vi "Main.vi"() -> ()   [LabVIEW 2024]
uses:
  <instrlib>/niScope/Acquire/Fetch/niScope Multi Fetch WDT.vi
panel:
  in  "Tab Control":T1(tab)
  in  "Scopes":refnum<k15>[](array[refnum])=["SCOPE1", "SCOPE2"] caption="resource name"
  in  "FGENs":refnum<k15>[](array[refnum])=["FGEN1", "FGEN2"] caption="Resource Name"
  out "Preparing NI-TClk":bool
  in  "Synchronization Method":enum32{"Manual", "T-Clk"}(radio)
  out "Phase Difference @ 10 MHz":dbl format="%#.2g °"
  out "Timing Diagram":digitalwaveform[](graph)
  in  "Stop":bool
  out "Waveform Graph":waveform(dbl)[](graph)
  # "Using NI-TClk to Align Sample Clocks and Improve Synchronization"
  # "Acquired Data"
  # "Time from Trigger to First Sample"
  # "Box Instruments: Cabled Connectivity"
  # "PXI: Integrated Connectivity"
  # "Hardware Configuration"
  # "Synchronization Method"
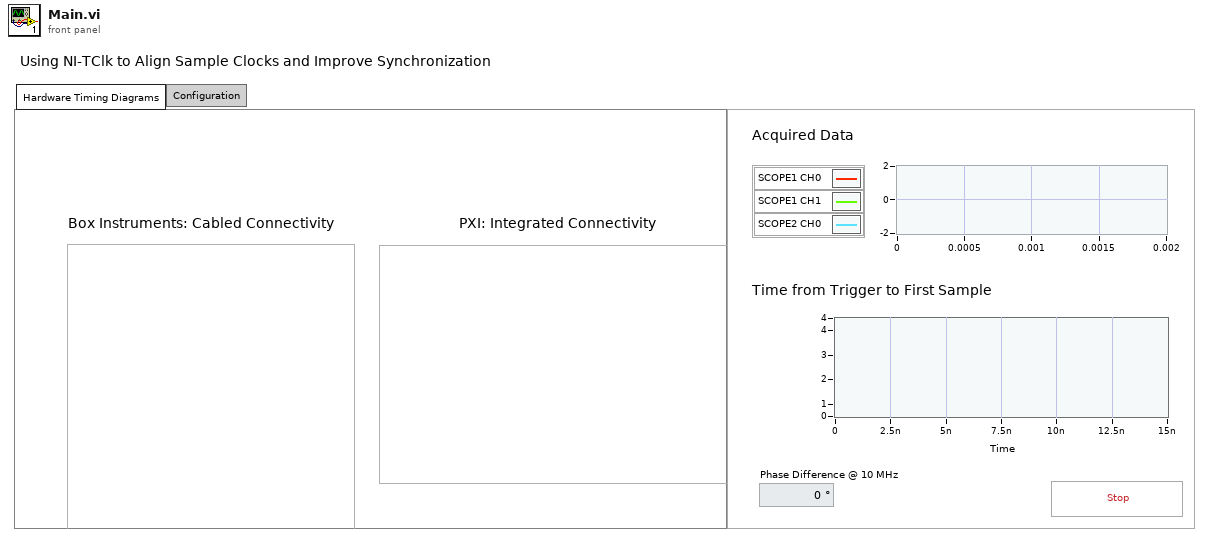
[diagram p1: front panel]
types:
  T1 = enum32{"Hardware Timing Diagrams", "Configuration"}
  T2 = cluster{"actualSamples":i32, "absoluteInitialX":dbl, "relativeInitialX":dbl, "xIncrement":dbl, "offset":dbl, "gain":dbl, "reserved1":dbl, "reserved2":dbl}[]
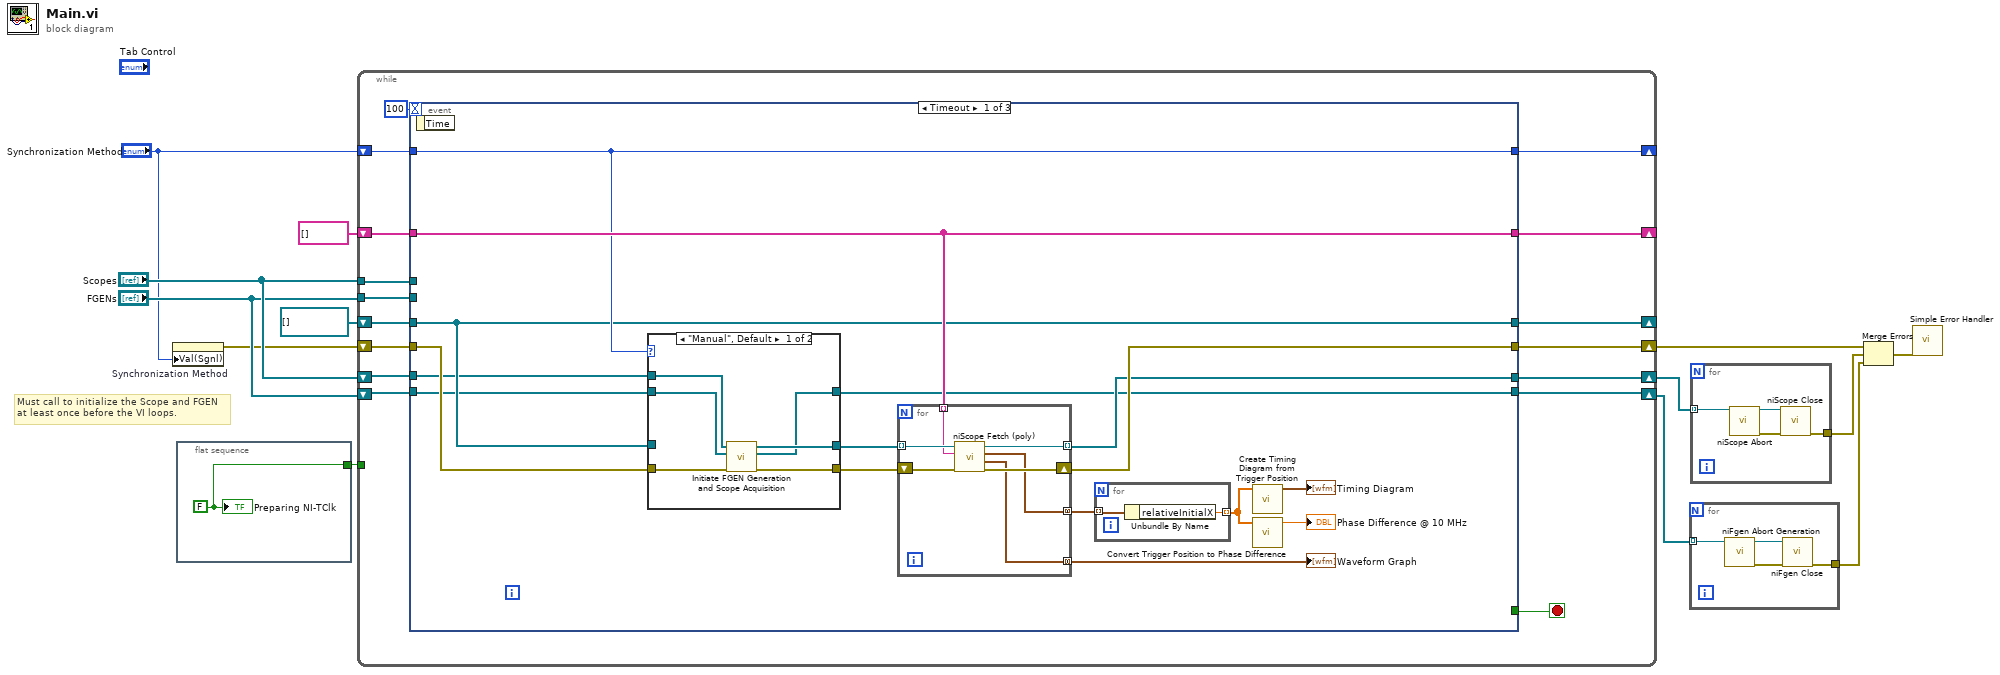
[diagram p0: block diagram]
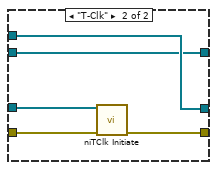
[diagram p2: hidden frame]
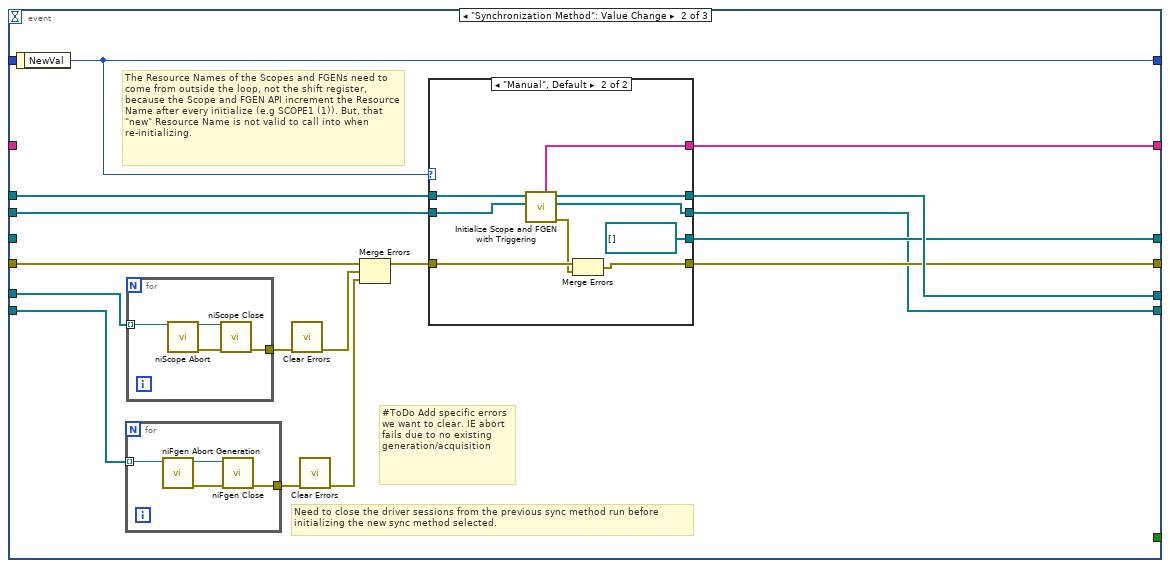
[diagram p3: hidden frame]
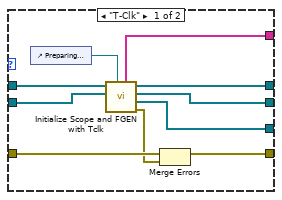
[diagram p4: hidden frame]
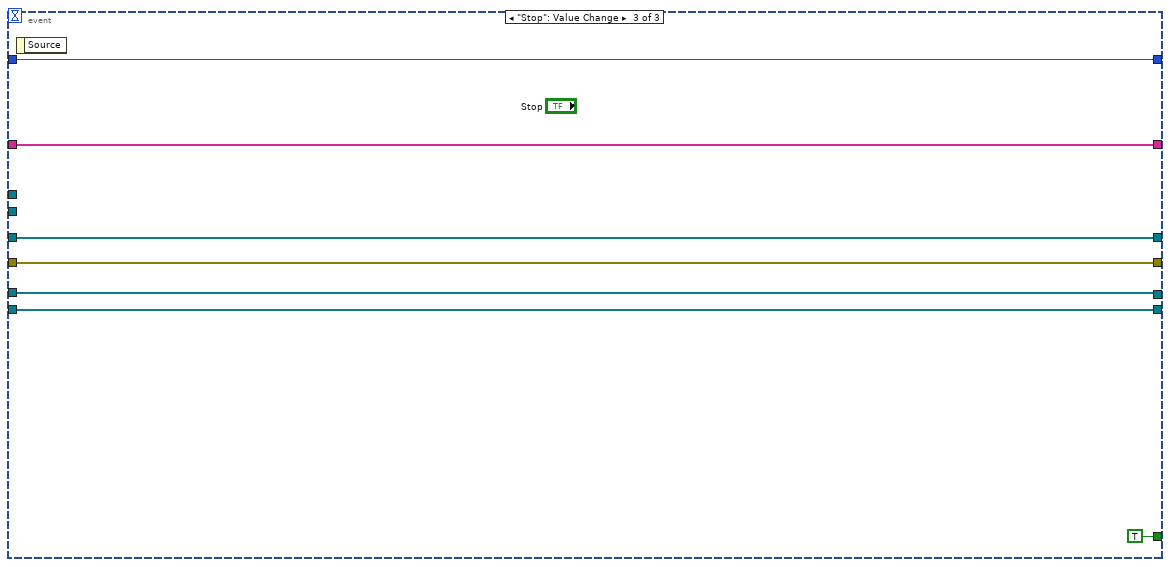
[diagram p5: hidden frame]
diagram:
  # "Must call to initialize the Scope and FGEN \nat least once before the VI loops."
  n1 = property on="Synchronization Method" class="RadioBtnsControl (strict)"("Val(Sgnl)"="Synchronization Method") -> (error out=w8:errorcluster)  [unwired: 2 in, 1 out]
  n2 = flat-sequence {
    tunnel: [w14] -> w9
    frame #0 {
      w14 = FALSE ("Preparing T-Clk")
      "Preparing NI-TClk" <- w14
    }
  }
  n3 = while {
    shift-right: [w28] -> _
    shift-left: "Synchronization Method" -> [w27]
    shift-right: [w24] -> _
    shift-left: string[] [] ("scope channels") -> [w20]
    shift-right: [w23] -> _
    shift-left: refnum<k20>[] [] ("Tclk Refs Array") -> [w21]
    shift-right: [w19] -> w5
    shift-left: w8 -> [w22]
    shift-right: [w16] -> w7
    shift-left: "Scopes" -> [w18]
    shift-right: [w15] -> w6
    shift-left: "FGENs" -> [w17]
    tunnel: w9 -> [_]
    tunnel: "Scopes" -> [w26]
    tunnel: "FGENs" -> [w25]
    stop <- w29 stop-if-true
    n4 = event shown="[0] Timeout" {
      selector: _ -> [_ _ _]
      dyn-events: _ -> [_ _ _]
      timeout: 100 -> [_ _ _]
      tunnel: [_ _ TRUE] -> w29
      tunnel: w25 -> [_ w77 _]
      tunnel: [w35 w82 w112] -> w28
      tunnel: w27 -> [w35 _ w112]
      tunnel: w26 -> [_ w78 _]
      tunnel: [w37 w81 w111] -> w16
      tunnel: [w36 w80 w115] -> w24
      tunnel: [w34 w79 w114] -> w23
      tunnel: w22 -> [w43 w74 w113]
      tunnel: w21 -> [w34 _ w114]
      tunnel: w20 -> [w36 _ w115]
      tunnel: [w38 w75 w113] -> w19
      tunnel: w18 -> [w33 w68 w111]
      tunnel: w17 -> [w32 w67 w110]
      tunnel: [w31 w69 w110] -> w15
      event Timeout {
        n5 = event-data() -> ()  [unwired: 1 in, 1 out]
        n6 = case shown="\"Manual\", Default" w35 {
          tunnel: [w49 w57] -> w42
          tunnel: w34 -> [_ w56]
          tunnel: w43 -> [w52 w55]
          tunnel: w33 -> [w48 w54]
          tunnel: w32 -> [w51 w53]
          tunnel: [w50 w54] -> w40
          tunnel: [w47 w53] -> w31
          frame "Manual", Default {
            n7 = call "Initiate FGEN Generation and Scope Acquisition.vi"("error in (no error)"=w52, "FGEN Resources in"=w51, "Scope Resources in"=w48) -> ("error out"=w49:errorcluster, "FGEN Resources out"=w47:refnum<k15>[], "Scope Resources out"=w50:refnum<k15>[])  [unwired: 6 in]
          }
          frame "T-Clk" {
            n8 = call <instrlib>:"niTClk Initiate.vi"("error in (no error)"=w55, "sessions"=w56) -> ("error out"=w57:errorcluster)  [unwired: 8 in, 1 out]
          }
        }
        n9 = for {
          tunnel: [w62] -> w44 mode=concatenating
          tunnel: [w61] -> w41 mode=concatenating
          shift-right: [w64] -> w38
          shift-left: w42 -> [w63]
          tunnel: w40 -> [w60] mode=indexing
          tunnel: w36 -> [w59] mode=indexing
          tunnel: [w58] -> w37 mode=indexing
          n10 = call-poly <instrlib>:"niScope Fetch (poly).vi"("error in"=w63, "channels"=w59, "instrument handle"=w60) -> ("error out"=w64:errorcluster, "wfm"=w62:waveform(dbl)[], "wfm info"=w61:T2, "instrument handle out"=w58:refnum<k15>)  [unwired: 5 in]
        }
        "Waveform Graph" <- w44
        n11 = for {
          tunnel: w41 -> [w66] mode=indexing
          tunnel: [w65] -> w39 mode=indexing
          n12 = Unbundle By Name(w66) -> ("relativeInitialX"=w65:dbl)
        }
        n13 = call "Create Timing Diagram from Trigger Position.vi"("Relative Trigger Position in"=w39) -> ("Timing Diagram"=→"Timing Diagram":digitalwaveform[])  [unwired: 10 in]
        n14 = call "Convert Trigger Position to Phase Difference.vi"("Relative Trigger Position in"=w39) -> ("Phase Difference"=→"Phase Difference @ 10 MHz":dbl)  [unwired: 10 in]
      }
      event "Synchronization Method": Value Change {
        # "The Resource Names of the Scopes and FGENs need to come from outside the loop, not the shift register, because the Scope and FGEN API increment the Resource Name after every initialize (e.g SCOPE1 (1)). But, that \"new\" Resource Name is not valid to call into when re-initializing."
        # "Need to close the driver sessions from the previous sync method run before\ninitializing the new sync method selected."
        # "#ToDo Add specific errors we want to clear. IE abort fails due to no existing generation/acquisition"
        n15 = event-data() -> ("NewVal"=w82:enum32{"Manual", "T-Clk"})  [unwired: 1 in]
        n16 = for {
          tunnel: w67 -> [w86] mode=indexing
          tunnel: [w85] -> w76
          n17 = call <instrlib>:"niFgen Abort Generation.vi"("Instrument Handle"=w86) -> ("error out"=w84:errorcluster, "Instrument Handle Out"=w83:refnum<k15>)  [unwired: 9 in]
          n18 = call <instrlib>:"niFgen Close.vi"("error in (no error)"=w84, "Instrument Handle"=w83) -> ("error out"=w85:errorcluster)  [unwired: 9 in]
        }
        n19 = for {
          tunnel: w68 -> [w90] mode=indexing
          tunnel: [w87] -> w70
          n20 = call <instrlib>:"niScope Abort.vi"("instrument handle"=w90) -> ("instrument handle out"=w89:refnum<k15>, "error out"=w88:errorcluster)  [unwired: 13 in]
          n21 = call <instrlib>:"niScope Close.vi"("instrument handle"=w89, "error in"=w88) -> ("error out"=w87:errorcluster)  [unwired: 13 in]
        }
        n22 = call <vilib>:"Clear Errors.vi"("error in (no error)"=w70) -> ("error out"=w72:errorcluster)  [unwired: 5 in, 1 out]
        n23 = call <vilib>:"Clear Errors.vi"("error in (no error)"=w76) -> ("error out"=w71:errorcluster)  [unwired: 5 in, 1 out]
        n24 = Merge Errors(w74, w72, w71) -> (w73:errorcluster)
        n25 = case shown="\"Manual\", Default" w82 {
          tunnel: w77 -> [w99 w108]
          tunnel: w78 -> [w100 w109]
          tunnel: [w98 w107] -> w81
          tunnel: [w97 w106] -> w69
          tunnel: [w96 w102] -> w80
          tunnel: [w95 refnum<k20>[] [] ("Tclk Refs Array")] -> w79
          tunnel: [w92 w104] -> w75
          tunnel: w73 -> [w94 w105]
          frame "T-Clk" {
            n26 = control-ref of="Preparing NI-TClk"() -> (w91:refnum<vi>)
            n27 = call "Initialize Scope and FGEN with Tclk.vi"("Tclk Boolean Ref"=w91, "FGEN Resources in"=w99, "Scope Resources in"=w100) -> ("error out"=w93:errorcluster, "Tclk Refs Array"=w95:refnum<k20>[], "FGEN Resources out"=w97:refnum<k15>[], "Scope Resources out"=w98:refnum<k15>[], "scope channels"=w96:string[])  [unwired: 4 in]
            n28 = Merge Errors(w94, w93) -> (w92:errorcluster)
          }
          frame "Manual", Default {
            n29 = call "Initialize Scope and FGEN with Triggering.vi"("FGEN Resources in"=w108, "Scope Resources in"=w109) -> ("error out"=w103:errorcluster, "FGEN Resources out"=w106:refnum<k15>[], "Scope Resources out"=w107:refnum<k15>[], "scope channels"=w102:string[])  [unwired: 6 in]
            n30 = Merge Errors(w105, w103) -> (w104:errorcluster)
          }
        }
      }
      event "Stop": Value Change {
        n31 = event-data() -> ()  [unwired: 1 in, 1 out]
      }
    }
  }
  n32 = for {
    tunnel: w6 -> [w120] mode=indexing
    tunnel: [w119] -> w3
    n33 = call <instrlib>:"niFgen Abort Generation.vi"("Instrument Handle"=w120) -> ("error out"=w118:errorcluster, "Instrument Handle Out"=w117:refnum<k15>)  [unwired: 9 in]
    n34 = call <instrlib>:"niFgen Close.vi"("error in (no error)"=w118, "Instrument Handle"=w117) -> ("error out"=w119:errorcluster)  [unwired: 9 in]
  }
  n35 = for {
    tunnel: w7 -> [w124] mode=indexing
    tunnel: [w121] -> w4
    n36 = call <instrlib>:"niScope Abort.vi"("instrument handle"=w124) -> ("instrument handle out"=w123:refnum<k15>, "error out"=w122:errorcluster)  [unwired: 13 in]
    n37 = call <instrlib>:"niScope Close.vi"("instrument handle"=w123, "error in"=w122) -> ("error out"=w121:errorcluster)  [unwired: 13 in]
  }
  n38 = Merge Errors(w5, w4, w3) -> (w2:errorcluster)
  n39 = call <vilib>:"Simple Error Handler.vi"("error in (no error)"=w2) -> ()  [unwired: 4 in, 5 out]
